vi "Simple Reader.vi"(8 "error in (no error)":errorcluster, 11 "Neocera Driver in":refnum<class "Neocera Driver.lvclass">) -> (0 "error out":errorcluster, 2 "Signals":dbl[](array[numeric]), 3 "Neocera Driver out":refnum<class "Neocera Driver.lvclass">)   [LabVIEW 2016, in "Neocera Driver.lvclass"]
uses:
  Neocera Driver.lvclass
  C:/github/NHMFL_Core/Libraries/Instruments/VISA Instrument/VISA Instrument.lvclass
  C:/github/NHMFL_Core/Libraries/Instruments/Temperature Controller Driver/Temperature Controller Driver.lvclass
  VISA Instrument/VISA Instrument.lvclass/VISA Instrument.ctl
  VISA Instrument/Read VISA resource.vi
  VISA Instrument/Write VISA resource.vi
  Temperature Controller Driver/Read T controller configuration.vi
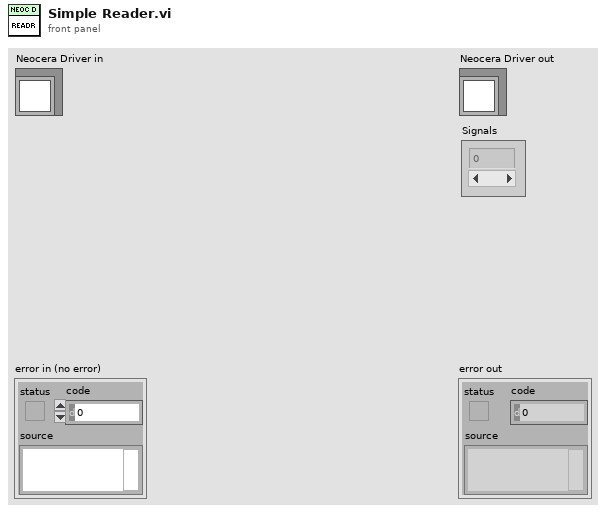
[diagram p1: front panel]
types:
  T1 = typedef "T controller configuration.ctl" = cluster{"Record Channels":string[], "Add raw signal":bool, "New set point":dbl}
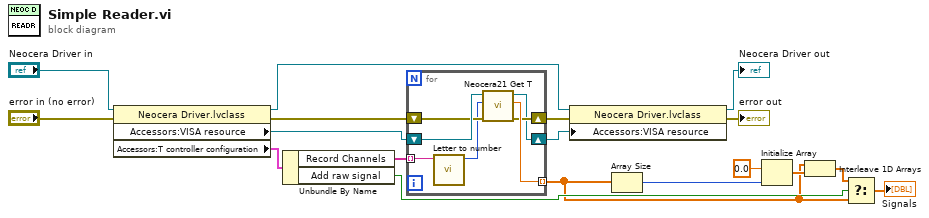
[diagram p0: block diagram]
diagram:
  n1 = property class="Neocera Driver.lvclass"(reference="Neocera Driver in", error in="error in (no error)") -> (reference out=w16:refnum<class "Neocera Driver.lvclass">, error out=w15:errorcluster, "Accessors:VISA resource"=w14:refnum<visa-resource-name>, "Accessors:T controller configuration"=w13:T1)
  n2 = Unbundle By Name(w13) -> ("Record Channels"=w12:string[], "Add raw signal"=w3:bool)
  n3 = for {
    tunnel: w12 -> [w20] mode=indexing
    tunnel: [w23] -> w2 mode=indexing
    shift-right: [w22] -> w18
    shift-left: w15 -> [w24]
    shift-right: [w21] -> w17
    shift-left: w14 -> [w25]
    n4 = call "Letter to number.vi"("String"=w20) -> ("Number"=w19:i32)  [unwired: 9 in, 1 out]
    n5 = call "Neocera21 Get T.vi"("error in (no error)"=w24, "Sensor"=w19, "VISA Resource Name"=w25) -> ("error out"=w22:errorcluster, "Temperature"=w23:dbl, "VISA Resource Name Out"=w21:refnum<visa-resource-name>)  [unwired: 5 in, 1 out]
  }
  n6 = property class="Neocera Driver.lvclass"(reference=w16, error in=w18, "Accessors:VISA resource"=w17) -> (reference out=→"Neocera Driver out":refnum<class "Neocera Driver.lvclass">, error out=→"error out":errorcluster)
  n7 = Array Size(array=w2) -> (size(s)=w7:i32)
  n8 = Initialize Array(0.0 ("element"), w7) -> (w5:dbl[])
  n9 = Interleave 1D Arrays(w2, w5) -> (w4:dbl[])
  n10 = Select(t=w4, s=w3, f=w2) -> (s? t:f=→"Signals":dbl[])
